vi "Control Panel Controller.vi"(8 "error in":errorcluster) -> ()   [LabVIEW 2020]
doc: "This VI executes continuously carrying out the current operation and responding to updates or new operations. It will often contain the timing or control code that is difficult to place directly in TeleOp. This VI generally opens all sensors and motors and isolates the rest of the robot code from knowing how the operations are carried out."
uses:
  <vilib>/Rock Robotics/WPI/Framework/Completion Status.ctl
  Control Panel Setpoints.ctl
  Control Panel Operations.ctl
  <vilib>/Rock Robotics/WPI/SafetyOutput/WPI_SafetyOutputConfigMenu.ctl
  <vilib>/Rock Robotics/Network Tables/NT Write Number.vi
panel:
  in  "Interactive Values":T1
  out "Current\nCmd":string
  in  "Buttons":cluster{"Execute Cmd":bool, "Abort Cmd":bool}
  out "Command Timing":cluster{"Start Time (ms)":u32, "Iterations":i32}
  out "Status":T3
  # "Tip: It may be helpful to observe inputs and sensor values.\nYou may also want to display tuning or debugging controls."
  # "Interactive Command: You may fill in the settings for a command\nand schedule it with the Execute button. You can observe and abort\nany command while fine tuning the code for the controller."
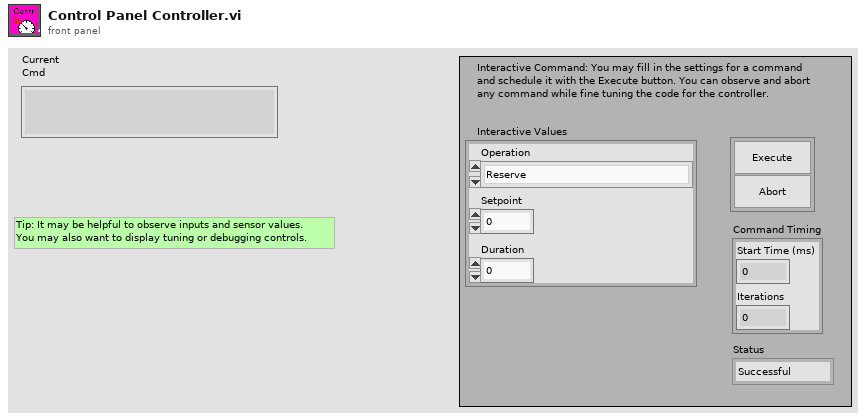
[diagram p1: front panel]
types:
  T1 = typedef "Control Panel Setpoints.ctl" = cluster{"Operation":T2, "Setpoint":dbl, "Duration":dbl}
  T2 = typedef "Control Panel Operations.ctl" = enum16{"Reserve", "Read Current", "Immediate", "for Time", "Stop"}
  T3 = typedef "Completion Status.ctl" = enum16{"Successful", "Aborted", "Incomplete"}
  T4 = typedef "WPI_SafetyOutputConfigMenu.ctl" = enum16{"Enable", "Disable"}
  T5 = typedef "WPI_MotorControlDeviceRef.ctl" = cluster{"DeviceStatus":errorcluster, "Type":T6, "PWM":cluster{"PWM Channel":T7, "DeadBand":T8}, "CAN":cluster{"Device Number":u8, "SetOutput VI Ref":variant, "GetOutput VI Ref":variant, "Enable VI Ref":variant, "Disable VI Ref":variant, "Data":variant}, "Invert":bool, "DIO PWM":cluster{"PWM \"Enable\" Channel":T7, "DIOChannel":T9, "PWM Rate":dbl}}
  T6 = typedef "WPI_MotorControlType.ctl" = enum16{"PWM", "CAN", "DIO PWM"}
  T7 = typedef "FPGA_DIOPWMChannel.ctl" = enum8{"PWM 0", "PWM 1", "PWM 2", "PWM 3", "PWM 4", "PWM 5", "PWM 6", "PWM 7", "PWM 8", "PWM 9", "PWM MXP 0", "PWM MXP 1", "PWM MXP 2", "PWM MXP 3", "PWM MXP 4", "PWM MXP 5", "PWM MXP 6", "PWM MXP 7", "PWM MXP 8", "PWM MXP 9", "Invalid"}
  T8 = typedef "WPI_PWMDeadband.ctl" = cluster{"Name":string, "maxPositivePwm":i32, "minPositivePwm":i32, "centerPwm":i32, "maxNegativePwm":i32, "minNegativePwm":i32, "angularRange":u16}
  T9 = typedef "FPGA_DIOChannel.ctl" = enum8{"DIO 0", "DIO 1", "DIO 2", "DIO 3", "DIO 4", "DIO 5", "DIO 6", "DIO 7", "DIO 8", "DIO 9", "DIO MXP 0", "DIO MXP 1", "DIO MXP 2", "DIO MXP 3", "DIO MXP 4", "DIO MXP 5", "DIO MXP 6", "DIO MXP 7", "DIO MXP 8", "DIO MXP 9", "DIO MXP 10", "DIO MXP 11", "DIO MXP 12", "DIO MXP 13", "DIO MXP 14", "DIO MXP 15", "SPI Port CS1", "SPI Port CS2", "SPI Port CS3", "SPI Port MISO", "SPI Port MOSI", "Invalid"}
  T10 = typedef "Command Status Info.ctl" = cluster{"Name":string, "Status":T3, "notifier out":T11}
  T11 = typedef "Completion Notifier.ctl" = refnum<notifier>
  T12 = cluster{"Current Command":T1, "Command Timing":cluster{"Start Time (ms)":u32, "Iterations":i32}, "Command Arguments":cluster{"Command Info":T10, "Description":string, "Default Command":T1, "queue out":refnum<queue>, "Subsystem Name":string}}
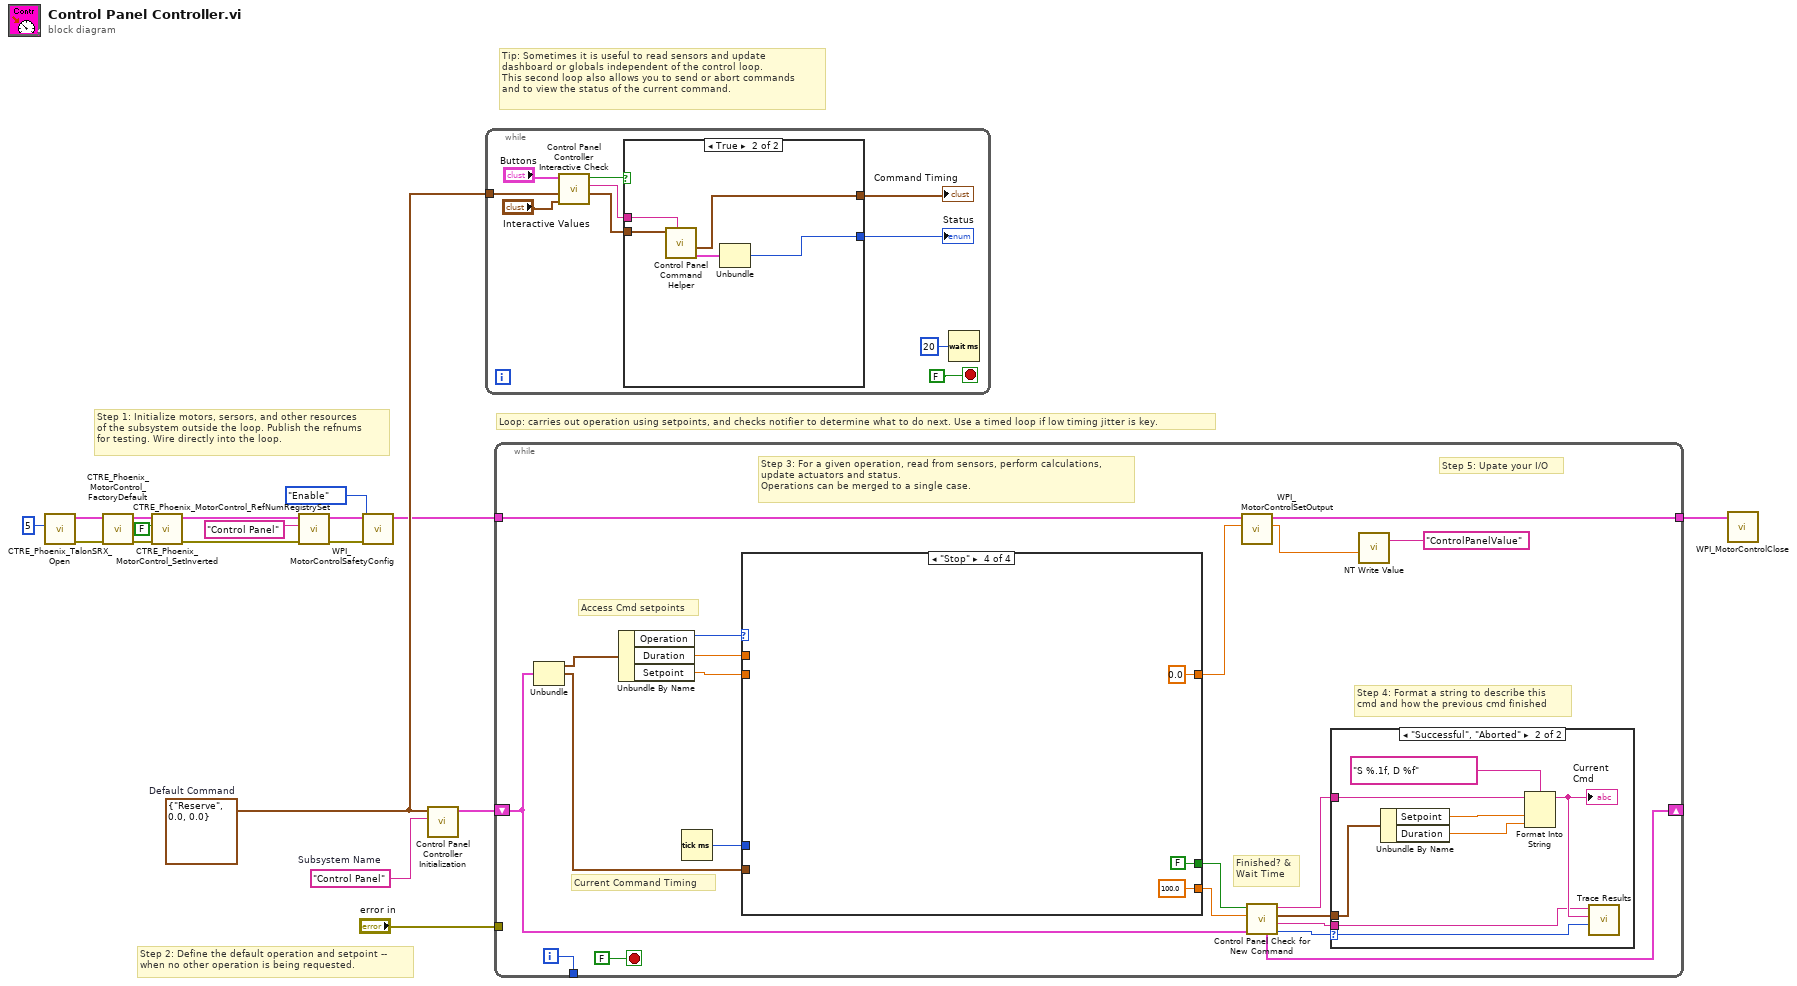
[diagram p0: block diagram]
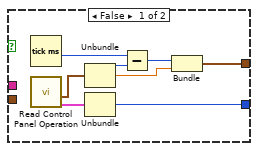
[diagram p2: hidden frame]
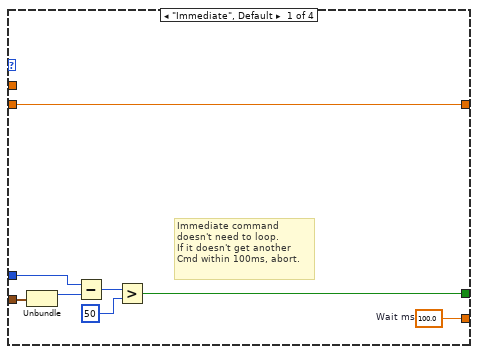
[diagram p4: hidden frame]
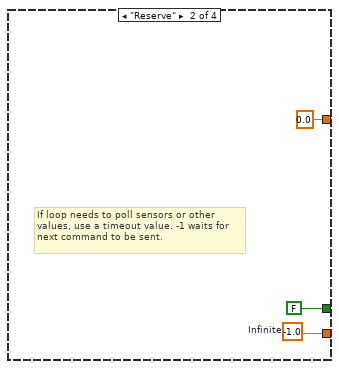
[diagram p5: hidden frame]
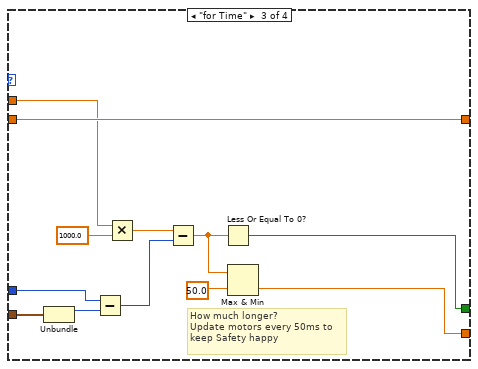
[diagram p6: hidden frame]
diagram:
  w15 = T1 {"Operation"=enum."Reserve", "Setpoint"=0.0, "Duration"=0.0}  # Default Command
  w16 = "Control Panel"  # Subsystem Name
  # "Tip: Sometimes it is useful to read sensors and update\ndashboard or globals independent of the control loop.\nThis second loop also allows you to send or abort commands\nand to view the status of the current command."
  # "Step 2: Define the default operation and setpoint --\nwhen no other operation is being requested."
  # "Step 1: Initialize motors, sersors, and other resources\nof the subsystem outside the loop. Publish the refnums\nfor testing. Wire directly into the loop."
  # "Loop: carries out operation using setpoints, and checks notifier to determine what to do next. Use a timed loop if low timing jitter is key."
  n1 = call <vilib>:"CTRE_Phoenix_TalonSRX_Open.vi"("Device Number"=u8 5) -> ("error out"=w14:errorcluster, "PhoenixMotorControlDevRef"=w13:T5)  [unwired: 9 in]
  n2 = call <vilib>:"CTRE_Phoenix_MotorControl_FactoryDefault.vi"("error in"=w14, "PhoenixMotorControlDevRef"=w13) -> ("error out"=w12:errorcluster, "PhoenixMotorControlDevRef"=w11:T5)  [unwired: 8 in]
  n3 = call <vilib>:"CTRE_Phoenix_MotorControl_SetInverted.vi"("error in (no error)"=w12, "Invert?"=FALSE, "PhoenixMotorControlDevRef"=w11) -> ("error out"=w10:errorcluster, "PhoenixMotorControlDevRef"=w9:T5)  [unwired: 7 in]
  n4 = call <vilib>:"CTRE_Phoenix_MotorControl_RefNumRegistrySet.vi"("error in (no error)"=w10, "refnum name"="Control Panel", "PhoenixMotorControlDevRef"=w9) -> ("error out"=w5:errorcluster, "PhoenixMotorControlDevRef"=w4:T5)  [unwired: 7 in]
  n5 = call <vilib>:"WPI_MotorControlSafetyConfig.vi"("error in (no error)"=w5, "mode"=WPI_SafetyOutputConfigMenu."Enable", "MotorControlDevRef"=w4) -> ("MotorControlDevRef"=w2:T5)  [unwired: 7 in, 1 out]
  n6 = call "Control Panel Controller Initialization.vi"("Subsystem Name"=w16, "Default Command"=w15) -> ("Current Command"=w17:T12)  [unwired: 9 in]
  n7 = while {
    tunnel: w15 -> [w25]
    stop <- FALSE stop-if-true
    n8 = call "Control Panel Controller Interactive Check.vi"("Interactive Command in"="Interactive Values", "Default Command"=w25, "Buttons"="Buttons") -> ("Interactive Command out"=w22:T1, "Trace String"=w23:string, "Schedule"=w24:bool)  [unwired: 6 in]
    n9 = case shown="True" w24 {
      tunnel: [w36 w41] -> w21
      tunnel: w22 -> [_ w39]
      tunnel: [w32 w37] -> w20
      tunnel: w23 -> [_ w40]
      frame False {
        n10 = Tick Count (ms)() -> (millisecond timer value=w31:u32)
        n11 = call "Read Control Panel Operation.vi"() -> ("Command Info"=w29:T10, "SubSystem Data"=w30:T1)  [unwired: 9 in, 1 out]
        n12 = Unbundle(w30) -> ("Operation"=w35:T2, "Setpoint"=w33:dbl)  [unwired: 1 out]
        n13 = Unbundle(w29) -> ("Status"=w36:T3)  [unwired: 2 out]
        n14 = Subtract(x=w31, y=w35) -> (x-y=w34:u32)
        n15 = Bundle(w34, "Setpoint"=w33) -> (w32:cluster{u32, "Setpoint":dbl})  [unwired: 1 in]
      }
      frame True {
        n16 = call "Control Panel Command Helper.vi"("Description"=w40, "SubSystem Data"=w39) -> ("Command Info Out"=w38:T10, "Command Timing"=w37:cluster{"Start Time (ms)":u32, "Iterations":i32})  [unwired: 7 in, 1 out]
        n17 = Unbundle(w38) -> ("Status"=w41:T3)  [unwired: 2 out]
      }
    }
    "Status" <- w21
    "Command Timing" <- w20
    n18 = Wait (ms)(milliseconds to wait=u32 20) -> ()  [unwired: 1 out]
  }
  n19 = while {
    shift-right: [w54] -> _
    shift-left: w17 -> [w47]
    tunnel: [w61] -> _
    tunnel: "error in" -> [_]
    tunnel: w2 -> [w46]
    tunnel: [w45] -> w1
    i -> [w61]
    stop <- FALSE stop-if-true
    # "Step 5: Upate your I/O"
    # "Step 4: Format a string to describe this\ncmd and how the previous cmd finished"
    # "Current Command Timing"
    # "Access Cmd setpoints"
    # "Finished? &\nWait Time"
    # "Step 3: For a given operation, read from sensors, perform calculations,\nupdate actuators and status.\nOperations can be merged to a single case."
    n20 = Unbundle(w47) -> ("Current Command"=w60:T1, "Command Timing"=w56:cluster{"Start Time (ms)":u32, "Iterations":i32})  [unwired: 1 out]
    n21 = Unbundle By Name(w60) -> ("Operation"=w59:T2, "Duration"=w58:dbl, "Setpoint"=w55:dbl)
    n22 = Tick Count (ms)() -> (millisecond timer value=w57:u32)
    n23 = case shown="\"Stop\"" w59 {
      tunnel: [w78 w81 w83 100.0 ("Infinite")] -> w52
      tunnel: [w72 FALSE ("ignore previous (F)") w82 FALSE ("ignore previous (F)")] -> w53
      tunnel: w56 -> [w74 _ w84 _]
      tunnel: w58 -> [_ _ w86 _]
      tunnel: w57 -> [w73 _ w85 _]
      tunnel: w55 -> [w71 _ w87 _]
      tunnel: [w71 0.0 ("Setpoint") w87 0.0 ("Setpoint")] -> w43
      frame "Immediate", Default {
        w78 = 100.0  # Wait ms
        # "Immediate command\ndoesn't need to loop.\nIf it doesn't get another\nCmd within 100ms, abort."
        n24 = Unbundle(w74) -> ("Start Time (ms)"=w77:u32)  [unwired: 1 out]
        n25 = Subtract(x=w73, y=w77) -> (x-y=w76:u32)
        n26 = Greater?(x=w76, y=u8 50 ("Left Motor")) -> (0:w72:bool)
      }
      frame "Reserve" {
        w81 = -1.0  # Infinite
        # "If loop needs to poll sensors or other\nvalues, use a timeout value. -1 waits for\nnext command to be sent."
      }
      frame "for Time" {
        # "How much longer?\nUpdate motors every 50ms to\nkeep Safety happy"
        n27 = Unbundle(w84) -> ("Start Time (ms)"=w90:u32)  [unwired: 1 out]
        n28 = Subtract(x=w85, y=w90) -> (x-y=w93:u32)
        n29 = Multiply(x=w86, y=1000.0) -> (x*y=w92:dbl)
        n30 = Subtract(x=w92, y=w93) -> (x-y=w89:dbl)
        n31 = Less Or Equal To 0?(x=w89) -> (x <= 0?=w82:bool)
        n32 = Max & Min(x=w89, y=50.0) -> (min(x,y)=w83:dbl)  [unwired: 1 out]
      }
      frame "Stop" {
      }
    }
    n33 = call <vilib>:"WPI_MotorControlSetOutput.vi"("Output"=w43, "MotorControlDevRef"=w46) -> ("Motor Output"=w44:dbl, "MotorControlDevRef"=w45:T5)  [unwired: 7 in, 1 out]
    n34 = call "Control Panel Check for New Command.vi"("Current Command"=w47, "Wait time (ms)"=w52, "Finished?"=w53) -> ("Completion"=w48:T3, "Subsystem Name"=w49:string, "Current Command"=w50:T1, "Initial Trace String"=w51:string, "NextCommand"=w54:T12)  [unwired: 4 in]
    n35 = case shown="\"Successful\", \"Aborted\"" w48 {
      selector: w48 -> [_ w70]
      tunnel: w51 -> [_ w66]
      tunnel: w50 -> [_ w67]
      tunnel: w49 -> [_ w63]
      frame "Incomplete", Default {
        # "Continuing current command"
      }
      frame "Successful", "Aborted" {
        # "Report and setup for next command"
        n36 = Unbundle By Name(w67) -> ("Setpoint"=w69:dbl, "Duration"=w64:dbl)
        n37 = Format Into String(format string="S %.1f, D %f", initial string=w66, w69, w64) -> (resulting string=w65:string)  [unwired: 1 in, 1 out]
        "Current\nCmd" <- w65
        n38 = call <vilib>:"Trace Results.vi"("Status of previous command"=w70, "Description"=w65, "Subsystem"=w63) -> ()  [unwired: 9 in]
      }
    }
    n39 = call-poly <vilib>:"NT Write Value.vi"("Numeric"=w44, "Name"="ControlPanelValue") -> ()  [unwired: 9 in, 1 out]
  }
  n40 = call <vilib>:"WPI_MotorControlClose.vi"("MotorControlDevRef"=w1) -> ()  [unwired: 10 in, 1 out]
